vi "Intake Process.vi"   [LabVIEW 2013]
uses:
  Intake Global.vi
types:
  T1 = typedef "WPI_RelayValue.ctl" = enum16{"Off", "On", "Forward", "Reverse"}
  T2 = typedef "WPI_SolenoidValue.ctl" = enum16{"Off", "On", "Forward", "Reverse"}
  T3 = cluster{"Arm State":bool, "Gripper In":bool, "Gripper Out":bool, "Gripper Execution":T1, "Arm Execution":T2, "Middle MS":bool, "Middle Stop":bool}
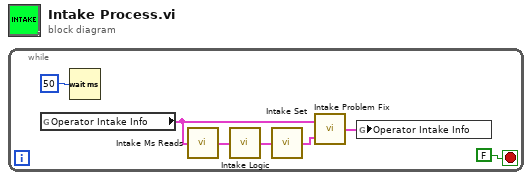
[diagram p0: block diagram]
diagram:
  n1 = while {
    stop <- FALSE stop-if-true
    n2 = global read "Intake Global.vi" "Operator Intake Info"() -> (w1:T3)
    n3 = Wait (ms)(milliseconds to wait=u32 50) -> ()  [unwired: 1 out]
    n4 = call "Intake Ms Reads.vi"("Operator Intake In"=w1) -> ("Operator Intake Out"=w2:T3)
    n5 = call "Intake Logic.vi"("Operator Intake In"=w2) -> ("Operator Intake Out"=w5:T3)
    n6 = call "Intake Set.vi"("Operator Intake In"=w5) -> ("Operator Intake Out"=w4:T3)
    n7 = call "Intake Problem Fix.vi"("Operator Intake Modified"=w4, "Operator Intake Original"=w1) -> ("Operator Intake Fixed"=w3:T3)
    n8 = global write "Intake Global.vi" "Operator Intake Info"(w3) -> ()
  }
